vi "update globals from exec.vi"(2 "Manual Power":dbl, 11 "PID exp exec":T2, 12 "exec.T mode":T1) -> (8 "Total elapsed time (s)":dbl=30.0, 15 "PID exp exec out":T2)   [LabVIEW 2019]
doc: "This subVI updates the bug global variables from the executive thread.\n\nPaul K Dixon\nP3600\nCSUSB Physics"
uses:
  typedefs/temp cont cluster.ctl
  typedefs/temp exec cluster.ctl
  typedefs/temp mode enum.ctl
  typedefs/temp indicator.ctl
  typedefs/temp cont utility.ctl
  typedefs/PID exec cluster.ctl
  typedefs/bug temp file info.ctl
  globals/Bug man temp globals.vi
panel:
  out "T cont out":T4 {"utility"."therm volt" format="%_6g"; "utility"."heat volt in" format="%_6g"; "utility"."heat volt out" format="%_6g"; "utility"."power out" format="%_6g"; "utility"."H Vmax" format="%_6g"; "exec"."man power" format="%_6g"; "T status"."Power" format="%_6g"; "T status"."Temp" format="%_6g"}
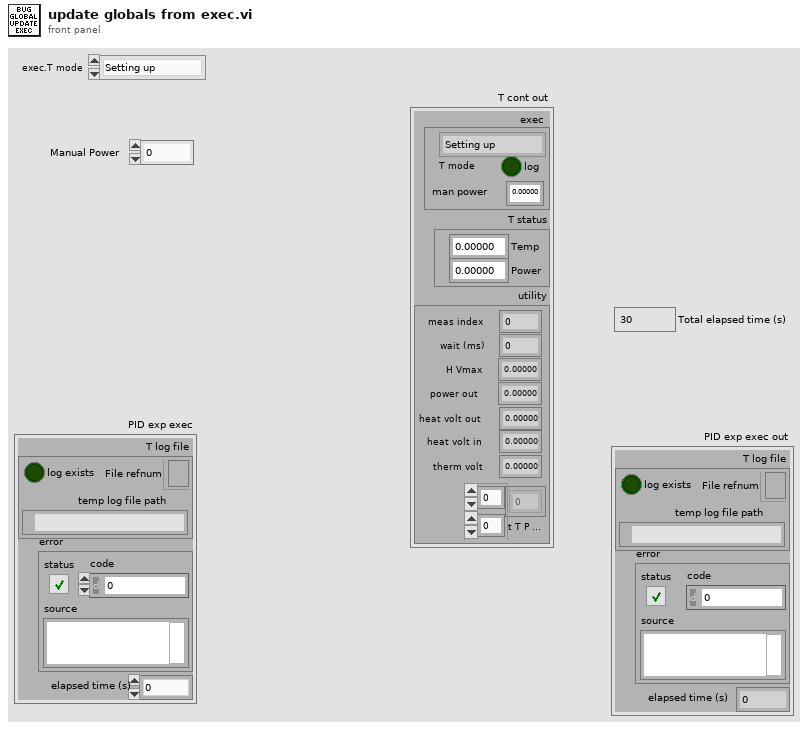
[diagram p1: front panel]
types:
  T1 = typedef "temp mode enum.ctl" = enum16{"Setting up", "Listening to exec", "Exit"}
  T2 = typedef "PID exec cluster.ctl" = cluster{"T log file":T3, "error":errorcluster, "elapsed time (s)":dbl}
  T3 = typedef "bug temp file info.ctl" = cluster{"log exists":bool, "File refnum":refnum<file>, "temp log file path":path}
  T4 = typedef "temp cont cluster.ctl" = cluster{"exec":T5, "T status":T6, "utility":T7}
  T5 = typedef "temp exec cluster.ctl" = cluster{"T mode":T1, "man power":dbl, "log":bool}
  T6 = typedef "temp indicator.ctl" = cluster{"Temp":dbl, "Power":dbl}
  T7 = typedef "temp cont utility.ctl" = cluster{"meas index":i32, "wait (ms)":i32, "H Vmax":dbl, "power out":dbl, "heat volt out":dbl, "heat volt in":dbl, "therm volt":dbl, "t T P hist":dbl[][]}
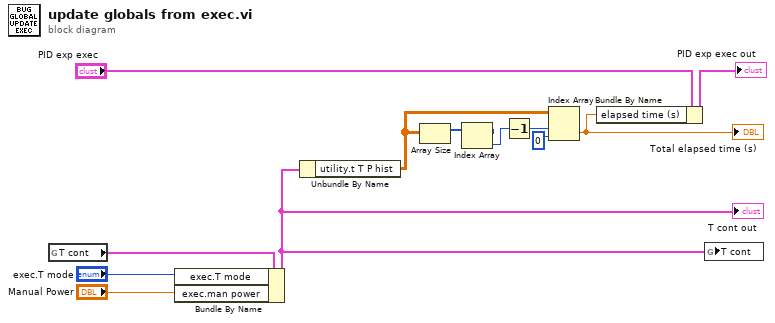
[diagram p0: block diagram]
diagram:
  n1 = global read "Bug man temp globals.vi" "T cont"() -> (w10:T4)
  n2 = Bundle By Name(cluster=w10, "exec.T mode"="exec.T mode", "exec.man power"="Manual Power") -> (w9:T4)
  "T cont out" <- w9
  n3 = Unbundle By Name(w9) -> ("utility.t T P hist"=w7:dbl[][])
  n4 = Array Size(array=w7) -> (size(s)=w4:i32[])
  n5 = Index Array(array=w4) -> (element=w3:i32)  [unwired: 1 in]
  n6 = Decrement(x=w3) -> (x-1=w5:i32)
  n7 = Index Array(array=w7, index (row)=w5, index (col)=0 ("disabled index (col)")) -> (element=w1:dbl)
  "Total elapsed time (s)" <- w1
  n8 = Bundle By Name(cluster="PID exp exec", "elapsed time (s)"=w1) -> (→"PID exp exec out":T2)
  n9 = global write "Bug man temp globals.vi" "T cont"(w9) -> ()
